vi "writeToXML.vi"(8 "error in (no error)":errorcluster, 10 "ClassLabel":string, 11 "GuideTargetConfiguration in":refnum<class "GuideTargetConfiguration.lvclass">) -> (0 "error out":errorcluster, 2 "XML out":string, 3 "GuideTargetConfiguration out":refnum<class "GuideTargetConfiguration.lvclass">)   [LabVIEW 2014, in "TCSDataDefinitions.lvlib" / "TCSCommand.lvlib" / "TargetConfiguration.lvlib" / "GuideTargetConfiguration.lvclass"]
uses:
  GuideTargetConfiguration.lvclass
  TargetConfiguration/TargetConfiguration.lvclass
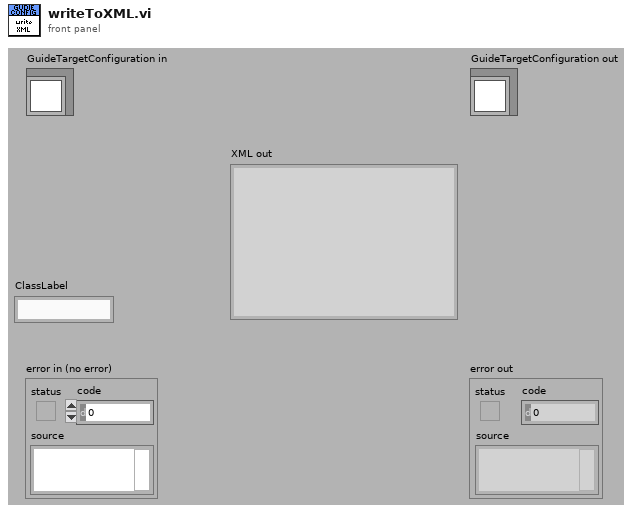
[diagram p1: front panel]
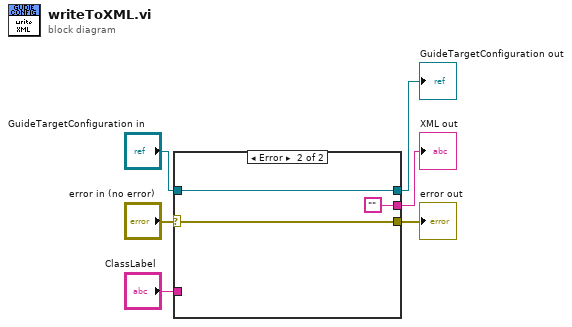
[diagram p0: block diagram]
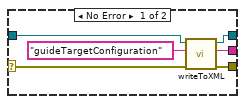
[diagram p2: hidden frame]
diagram:
  n1 = case shown="Error" "error in (no error)" {
    selector: "error in (no error)" -> [w12 w15]
    tunnel: [w11 w15] -> w5
    tunnel: [w9 w14] -> w3
    tunnel: "GuideTargetConfiguration in" -> [w10 w14]
    tunnel: "ClassLabel" -> [_ _]
    tunnel: [w8 ""] -> w1
    frame No Error {
      n2 = call-parent "writeToXML.vi"("error in (no error)"=w12, "classLabel"="guideTargetConfiguration", "TargetConfiguration in"=w10) -> ("error out"=w11:errorcluster, "XML out"=w8:string, "TargetConfiguration out"=w9:refnum<class "GuideTargetConfiguration.lvclass">)  [unwired: 6 in]
    }
    frame Error {
    }
  }
  "error out" <- w5
  "GuideTargetConfiguration out" <- w3
  "XML out" <- w1
